vi "SnoReturnCatapult[Conflict].vi"   [LabVIEW 2013]
uses:
  <vilib>/Rock Robotics/WPI/Solenoid/WPI_SolenoidValue.ctl
  <vilib>/Rock Robotics/WPI/Solenoid/WPI_SolenoidSetEnum.vi
types:
  T1 = typedef "WPI_SolenoidValue.ctl" = enum16{"Off", "On", "Forward", "Reverse"}
  T2 = typedef "WPI_SolenoidDevRef.ctl" = cluster{"DevStatus":errorcluster, "Solenoid Module":T3, "Forward Solenoid Channel":T4, "Reverse Solenoid Channel":T4}
  T3 = typedef "FPGA_TypedefSolenoidModule.ctl" = enum16{"Solenoid Module 1", "Solenoid Module 2"}
  T4 = typedef "WPI_SolenoidChannel.ctl" = enum8{"Solenoid 1", "Solenoid 2", "Solenoid 3", "Solenoid 4", "Solenoid 5", "Solenoid 6", "Solenoid 7", "Solenoid 8", "Invalid"}
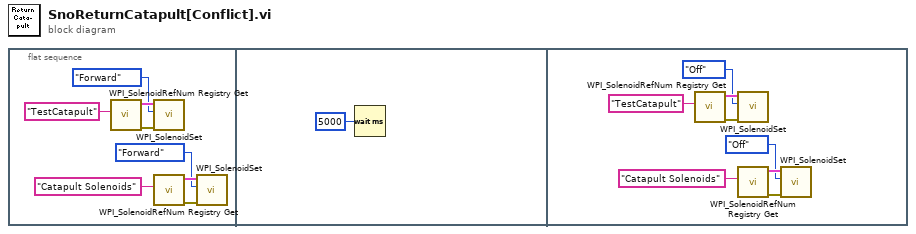
[diagram p0: block diagram]
diagram:
  n1 = flat-sequence {
    frame #0 {
      n2 = call <vilib>:"WPI_SolenoidRefNum Registry Get.vi"("refnum name"="TestCatapult") -> ("error out"=w7:errorcluster, "SolenoidDevRef"=w8:T2)  [unwired: 9 in]
      n3 = call-poly <vilib>:"WPI_SolenoidSet.vi"("error in (no error)"=w7, "Value"=WPI_SolenoidValue."Forward", "SolenoidDevRef"=w8) -> ()  [unwired: 7 in, 2 out]
      n4 = call <vilib>:"WPI_SolenoidRefNum Registry Get.vi"("refnum name"="Catapult Solenoids") -> ("error out"=w4:errorcluster, "SolenoidDevRef"=w3:T2)  [unwired: 9 in]
      n5 = call-poly <vilib>:"WPI_SolenoidSet.vi"("error in (no error)"=w4, "Value"=WPI_SolenoidValue."Forward", "SolenoidDevRef"=w3) -> ()  [unwired: 7 in, 2 out]
    }
    frame #1 {
      n6 = Wait (ms)(milliseconds to wait=u32 5000) -> ()  [unwired: 1 out]
    }
    frame #2 {
      n7 = call <vilib>:"WPI_SolenoidRefNum Registry Get.vi"("refnum name"="TestCatapult") -> ("error out"=w16:errorcluster, "SolenoidDevRef"=w17:T2)  [unwired: 9 in]
      n8 = call-poly <vilib>:"WPI_SolenoidSet.vi"("error in (no error)"=w16, "Value"=WPI_SolenoidValue."Off", "SolenoidDevRef"=w17) -> ()  [unwired: 7 in, 2 out]
      n9 = call <vilib>:"WPI_SolenoidRefNum Registry Get.vi"("refnum name"="Catapult Solenoids") -> ("error out"=w13:errorcluster, "SolenoidDevRef"=w12:T2)  [unwired: 9 in]
      n10 = call-poly <vilib>:"WPI_SolenoidSet.vi"("error in (no error)"=w13, "Value"=WPI_SolenoidValue."Off", "SolenoidDevRef"=w12) -> ()  [unwired: 7 in, 2 out]
    }
  }
